vi "HiPot_IDN.vi"(8 "error in (no error)":errorcluster, 11 "VISA Refnum in":refnum<visa-resource-name>) -> (0 "error out":errorcluster, 2 "read buffer":string, 3 "new?":bool)   [LabVIEW 2013]
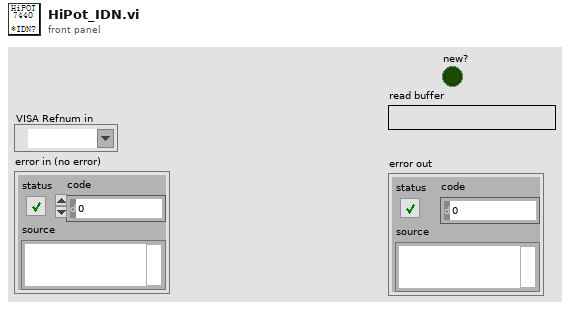
[diagram p1: front panel]
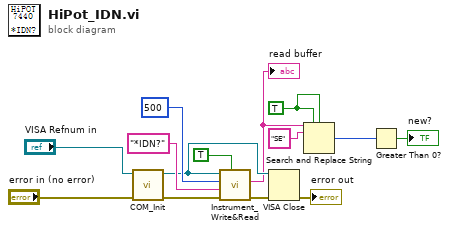
[diagram p0: block diagram]
diagram:
  w4 = TRUE ("replace all? (F)")
  n1 = call "COM_Init.vi"("error in (no error)"="error in (no error)", "VISA Refnum in"="VISA Refnum in") -> ("error out"=w7:errorcluster, "VISA Refnum out"=w9:refnum<visa-resource-name>)  [unwired: 8 in]
  n2 = call "Instrument_Write&Read.vi"("Read?"=TRUE, "Error In"=w7, "CMD"="*IDN?", "wait ms"=500, "PORT"=w9) -> ("Error Out"=w10:errorcluster, "read buffer"=w5:string)  [unwired: 5 in]
  "read buffer" <- w5
  n3 = VISA Close(VISA resource name=w9, error in (no error)=w10) -> (error out=→"error out":errorcluster)
  n4 = Search and Replace String(replace all?=w4, case sensitive?=w4, input string=w5, search string="SE") -> (number of replacements=w2:i32)  [unwired: 4 in, 3 out]
  n5 = Greater Than 0?(x=w2) -> (x > 0?=→"new?":bool)
